vi "EnQ Helper Loop Q DVR.vi"() -> ()   [LabVIEW 2021, in "Helper Loop.lvclass"]
uses:
  Helper Loop.lvclass
panel:
  out "error out":errorcluster
  out "Helper Loop Q DVR":refnum<data-value>
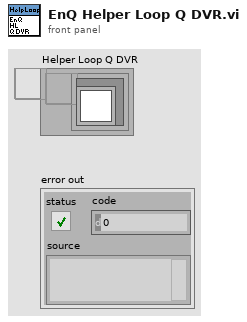
[diagram p1: front panel]
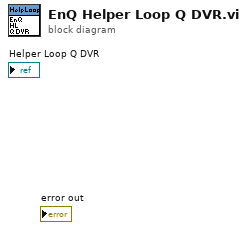
[diagram p0: block diagram]
diagram:
